vi "direct_kinematics.vi"(0 "j4":dbl, 1 "j5":dbl, 2 "j6":dbl, 3 "l5":dbl, 4 "l4":dbl, 5 "l3":dbl, 6 "j3":dbl, 7 "l2":dbl, 8 "j2":dbl, 9 "l1":dbl, 10 "j1":dbl, 11 "base":dbl) -> (13 "Translation Matrix":T1, 14 "X":dbl, 15 "Y":dbl, 16 "Z":dbl, 17 "RX":dbl, 18 "RY":dbl, 19 "RZ":dbl)   [LabVIEW 2019]
uses:
  <vilib>/Analysis/Matrix/Datatypes/RealMatrix.ctl
  <vilib>/Analysis/baseanly.llb/Real A x B.vi
  <vilib>/Analysis/baseanly.llb/A x Vector.vi
  <vilib>/Analysis/baseanly.llb/Real Inverse Matrix.vi
  <vilib>/Analysis/NI_AALBase.lvlib
  <vilib>/robotics/Kinematics/NI_Kinematics.lvlib
  <vilib>/Analysis/Matrix/NI_Matrix.lvlib
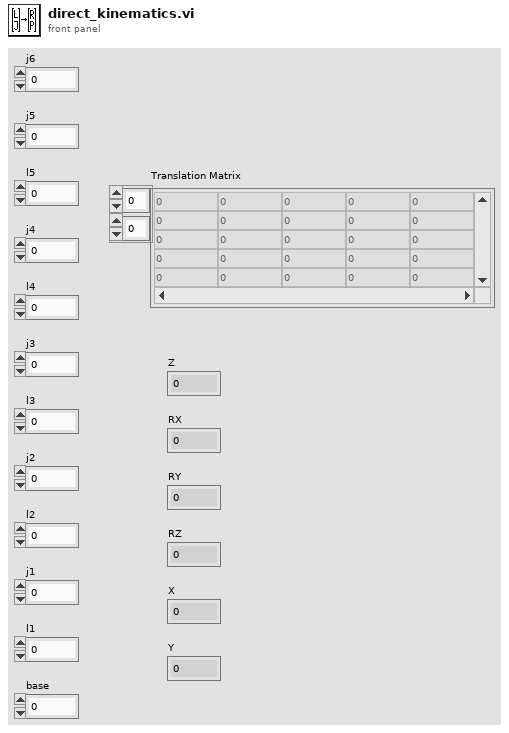
[diagram p1: front panel]
types:
  T1 = typedef "NI_Matrix.lvlib/RealMatrix.ctl" = dbl[][]
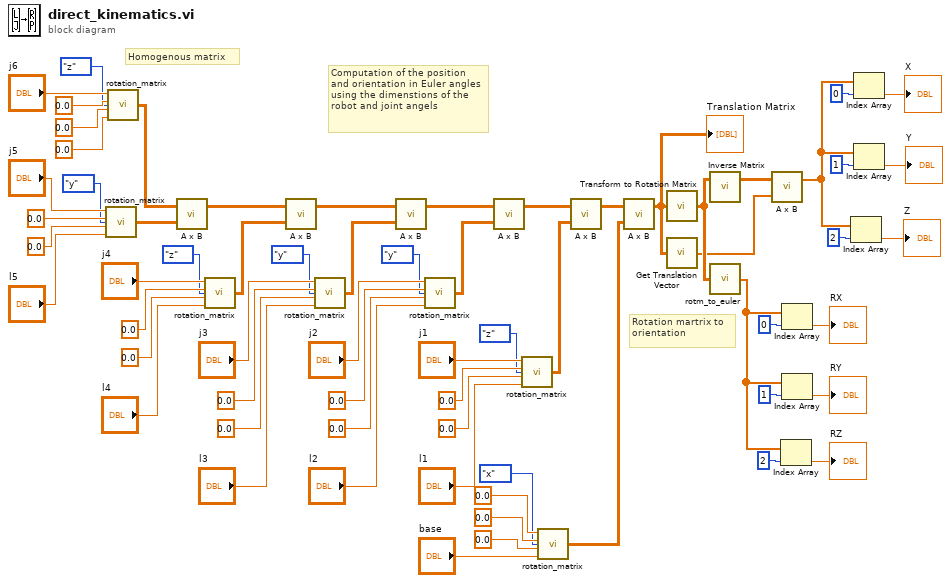
[diagram p0: block diagram]
diagram:
  # "Rotation martrix to orientation"
  # "Homogenous matrix"
  # "Computation of the position and orientation in Euler angles using the dimenstions of the robot and joint angels"
  n1 = call "rotation_matrix.vi"("Rotation"="j5", "Translation X"=0.0, "Translation Y"=0.0, "Translation Z"="l5", "Enum"=enum16{"x", "y", "z"}."y") -> ("Real Matrix"=w36:T1)
  n2 = call "rotation_matrix.vi"("Rotation"="j6", "Translation X"=0.0, "Translation Y"=0.0, "Translation Z"=0.0, "Enum"=enum16{"x", "y", "z"}."z") -> ("Real Matrix"=w35:T1)
  n3 = call-poly <vilib>:"A x B.vi"("B"=w36, "A"=w35) -> ("A x B"=w37:T1)  [unwired: 1 out]
  n4 = call "rotation_matrix.vi"("Rotation"="j4", "Translation X"=0.0, "Translation Y"=0.0, "Translation Z"="l4", "Enum"=enum16{"x", "y", "z"}."z") -> ("Real Matrix"=w38:T1)
  n5 = call-poly <vilib>:"A x B.vi"("B"=w38, "A"=w37) -> ("A x B"=w39:T1)  [unwired: 1 out]
  n6 = call "rotation_matrix.vi"("Rotation"="j3", "Translation X"=0.0, "Translation Y"=0.0, "Translation Z"="l3", "Enum"=enum16{"x", "y", "z"}."y") -> ("Real Matrix"=w40:T1)
  n7 = call-poly <vilib>:"A x B.vi"("B"=w40, "A"=w39) -> ("A x B"=w42:T1)  [unwired: 1 out]
  n8 = call "rotation_matrix.vi"("Rotation"="j2", "Translation X"=0.0, "Translation Y"=0.0, "Translation Z"="l2", "Enum"=enum16{"x", "y", "z"}."y") -> ("Real Matrix"=w41:T1)
  n9 = call-poly <vilib>:"A x B.vi"("B"=w41, "A"=w42) -> ("A x B"=w43:T1)  [unwired: 1 out]
  n10 = call "rotation_matrix.vi"("Rotation"="j1", "Translation X"=0.0, "Translation Y"=0.0, "Translation Z"="l1", "Enum"=enum16{"x", "y", "z"}."z") -> ("Real Matrix"=w44:T1)
  n11 = call "rotation_matrix.vi"("Rotation"=0.0, "Translation X"=0.0, "Translation Y"=0.0, "Translation Z"="base", "Enum"=enum16{"x", "y", "z"}."x") -> ("Real Matrix"=w46:T1)
  n12 = call-poly <vilib>:"A x B.vi"("B"=w44, "A"=w43) -> ("A x B"=w45:T1)  [unwired: 1 out]
  n13 = call-poly <vilib>:"A x B.vi"("B"=w46, "A"=w45) -> ("A x B"=w34:T1)  [unwired: 1 out]
  "Translation Matrix" <- w34
  n14 = call <vilib>:"Transform to Rotation Matrix.vi"("transform"=w34) -> ("rotation matrix"=w48:T1)
  n15 = call <vilib>:"Get Translation Vector.vi"("transform"=w34) -> ("translation vector"=w33:dbl[])
  n16 = call-poly <vilib>:"Inverse Matrix.vi"("Input Matrix"=w48) -> ("Inverse Matrix"=w47:T1)  [unwired: 1 in, 1 out]
  n17 = call "rotm_to_euler.vi"("Rotation Matrix"=w48) -> ("Orientation XYZ"=w52:dbl[])
  n18 = call-poly <vilib>:"A x B.vi"("Vector"=w33, "A"=w47) -> ("A x Vector"=w59:dbl[])  [unwired: 1 out]
  n19 = Index Array(array=w52, index=2) -> (element=→"RZ":dbl)
  n20 = Index Array(array=w52, index=0) -> (element=→"RX":dbl)
  n21 = Index Array(array=w52, index=1) -> (element=→"RY":dbl)
  n22 = Index Array(array=w59, index=2) -> (element=→"Z":dbl)
  n23 = Index Array(array=w59, index=0) -> (element=→"X":dbl)
  n24 = Index Array(array=w59, index=1) -> (element=→"Y":dbl)
